vi "Read mutex.vi"(8 "error in (no error)":errorcluster, 11 "Network Master in":refnum<class "Network Master.lvclass">) -> (0 "error out":errorcluster, 2 "mutex":refnum<data-value>, 3 "Network Master out":refnum<class "Network Master.lvclass">)   [LabVIEW 2021, in "Network Master.lvclass"]
uses:
  Network Master.lvclass
  Network Master.lvclass/Network Master.ctl
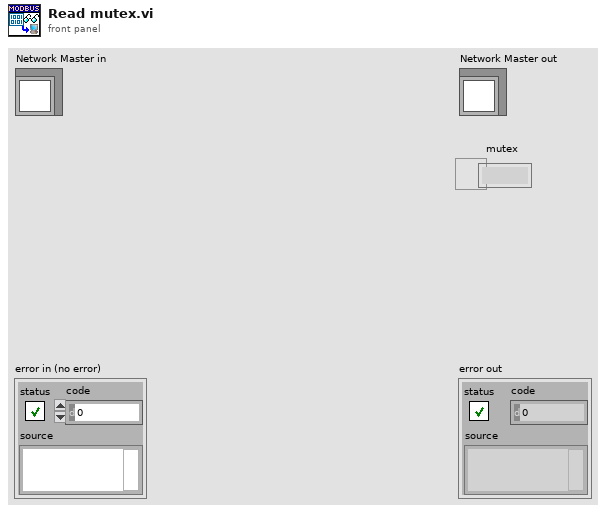
[diagram p1: front panel]
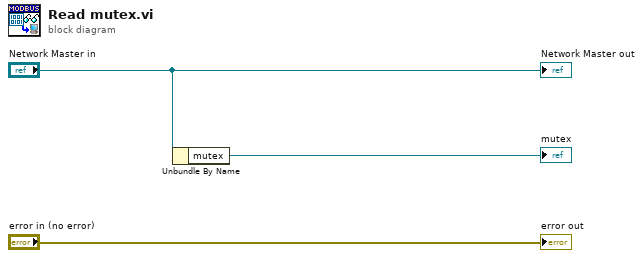
[diagram p0: block diagram]
diagram:
  n1 = Unbundle By Name("Network Master in") -> ("mutex"=→"mutex":refnum<data-value>)
  "error out" <- "error in (no error)"
  "Network Master out" <- "Network Master in"
